vi "Align Position Convert.vi"(8 "error in":errorcluster, 9 "Resolution":T1, 10 "Focus Center":cluster{"x":sgl, "y":sgl}, 11 "Position in":dbl[](array[numeric])) -> (0 "error out":errorcluster, 3 "Position out":dbl[](array[numeric]))   [LabVIEW 2019, in "Image.lvlib"]
uses:
  Image.lvlib
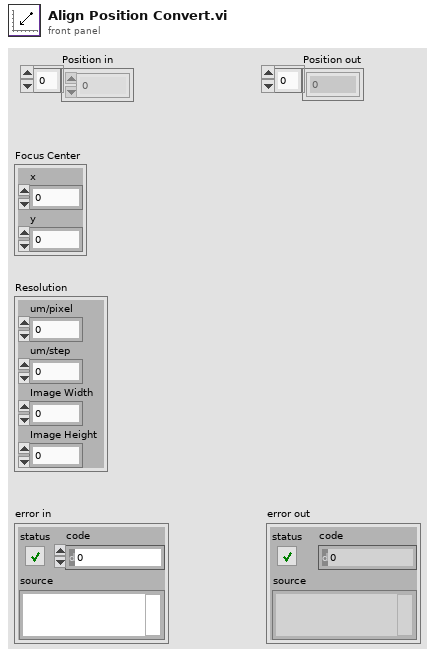
[diagram p1: front panel]
types:
  T1 = cluster{"um/pixel":dbl, "um/step":dbl, "Image Width":dbl, "Image Height":dbl}
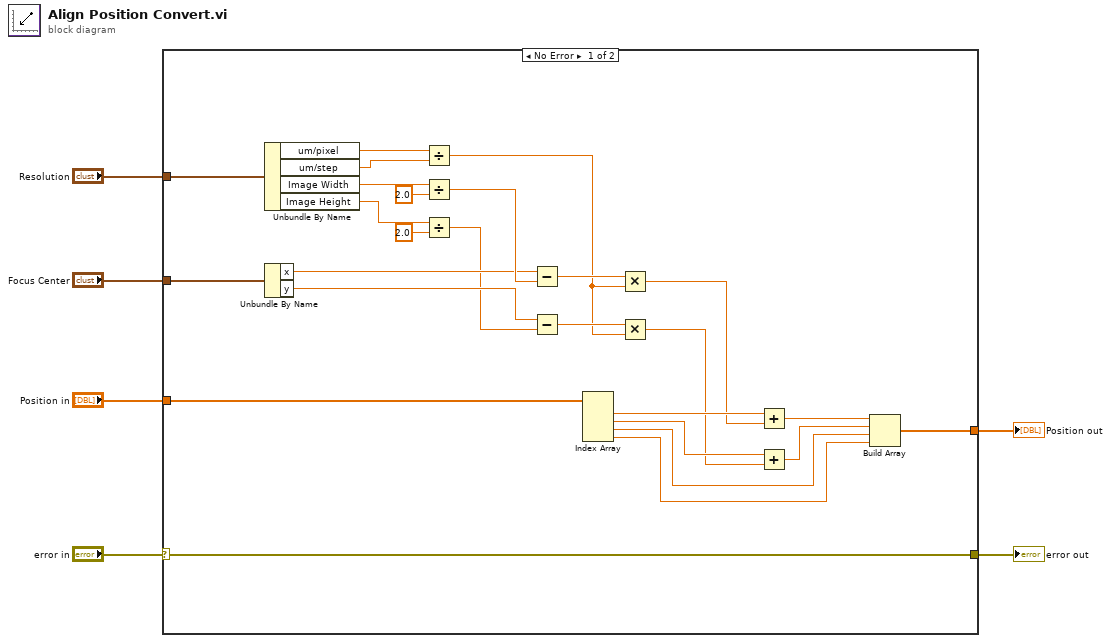
[diagram p0: block diagram]
diagram:
  n1 = case shown="No Error" "error in" {
    selector: "error in" -> [w11 w34]
    tunnel: "Resolution" -> [w32 _]
    tunnel: "Focus Center" -> [w31 _]
    tunnel: "Position in" -> [w21 w33]
    tunnel: [w12 w33] -> w3
    tunnel: [w11 w34] -> w1
    frame No Error {
      n2 = Unbundle By Name(w32) -> ("um/pixel"=w26:dbl, "um/step"=w25:dbl, "Image Width"=w30:dbl, "Image Height"=w28:dbl)
      n3 = Unbundle By Name(w31) -> ("x"=w9:sgl, "y"=w8:sgl)
      n4 = Divide(x=w26, y=w25) -> (x/y=w22:dbl)
      n5 = Divide(x=w30, y=2.0) -> (x/y=w10:dbl)
      n6 = Divide(x=w28, y=2.0) -> (x/y=w7:dbl)
      n7 = Subtract(x=w9, y=w10) -> (x-y=w24:dbl)
      n8 = Subtract(x=w8, y=w7) -> (x-y=w23:dbl)
      n9 = Index Array(array=w21) -> (element #1=w20:dbl, element #2=w18:dbl, element #3=w14:dbl, element #4=w13:dbl)  [unwired: 4 in]
      n10 = Multiply(x=w24, y=w22) -> (x*y=w19:dbl)
      n11 = Multiply(x=w23, y=w22) -> (x*y=w17:dbl)
      n12 = Add(x=w20, y=w19) -> (x+y=w16:dbl)
      n13 = Add(x=w18, y=w17) -> (x+y=w15:dbl)
      n14 = Build Array(w16, w15, w14, w13) -> (w12:dbl[])
    }
    frame Error {
    }
  }
  "Position out" <- w3
  "error out" <- w1
